vi "Torque Page.vi"(8 "error in (no error)":errorcluster, 11 "Node Ptr":T5 format="%.0x") -> (0 "error out":errorcluster)   [LabVIEW 2010, in "PXIe-433x Custom Device.lvlib"]
uses:
  PXIe-433x Custom Device.lvlib
  <vilib>/NI Veristand/Custom Device API/Custom Device Item Ref.ctl
  Generic Bridge Information.ctl
  Torque Scaling Information.ctl
  Max Value.ctl
  Min Value.ctl
  Board Info for checking settings.ctl
  Scale Type.ctl
  Sensor Type.ctl
  Global.vi
  <vilib>/NI VeriStand/Custom Device API/Get Item Property (Variant).vi
  <vilib>/NI VeriStand/Custom Device API/Get Item Property (Double).vi
  <vilib>/NI Veristand/Custom Device API/Set Item Property (Variant).vi
  <vilib>/NI Veristand/Custom Device API/Set Item Property (Double).vi
  <vilib>/NI Veristand/Custom Device API/Custom Device API.lvlib
panel:
  in  "Board Info for checking":T1
  in  "Minimum Value":T2=-0.05 caption="lb-in"
  in  "Maximum Value":T3=0.05 caption="lb-in"
  out "Error Description":string
  out "Tab Control":enum32{"No Error", "No Check", "Error"}(tab)
  out "Valid":bool=TRUE
  in  "No Error Check Details":bool
  out "No Check":bool=TRUE
  in  "Error Details":bool
  in  "stop":bool
  out "Valid Configuration?":bool
  in  "bridge information":T4={"bridge configuration"=10182, "voltage excitation source"=10200, "voltage excitation value"=2.5, "nominal bridge resistance"=350.0} {"voltage excitation source" items=["Internal"=10200, "External"=10167]; "bridge configuration" items=["Full Bridge"=10182, "Half Bridge"=10187, "Quarter Bridge"=10270]}
  in  "scaling information":T6={"first electrical value"=0.0, "second electrical value"=2.0, "electrical units"=15897, "first physical value"=0.0, "second physical value"=100.0, "physical units"=15883} {"physical units" items=["Nm"=15881, "oz-in"=15882, "lb-in"=15883, "lb-ft"=15884]; "electrical units" items=["Volts/Volt"=15896, "mVolts/Volt"=15897]}
  # "No Error"
  # "No Error"
  # "No Error Check"
  # "No Error Check"
  # "Error!"
  # "Error!"
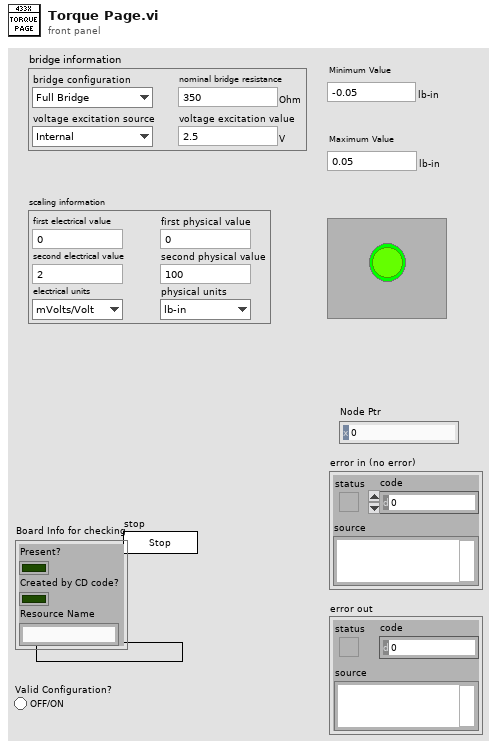
[diagram p1: front panel]
types:
  T1 = typedef "PXIe-433x Custom Device.lvlib/Board Info for checking settings.ctl" = cluster{"Present?":bool, "Created by CD code?":bool, "Resource Name":string}
  T2 = typedef "PXIe-433x Custom Device.lvlib/Min Value.ctl" = dbl
  T3 = typedef "PXIe-433x Custom Device.lvlib/Max Value.ctl" = dbl
  T4 = typedef "PXIe-433x Custom Device.lvlib/Generic Bridge Information.ctl" = cluster{"bridge configuration":i32, "voltage excitation source":i32, "voltage excitation value":dbl, "nominal bridge resistance":dbl}
  T5 = typedef "Custom Device API.lvlib/Custom Device Item Ref.ctl" = u64
  T6 = typedef "PXIe-433x Custom Device.lvlib/Torque Scaling Information.ctl" = cluster{"first electrical value":dbl, "second electrical value":dbl, "electrical units":i32, "first physical value":dbl, "second physical value":dbl, "physical units":i32}
  T7 = typedef "PXIe-433x Custom Device.lvlib/Scale Type.ctl" = enum16{"Linear", "Table", "Polynomial"}
  T8 = typedef "PXIe-433x Custom Device.lvlib/Sensor Type.ctl" = enum16{"Strain", "Force", "Pressure", "Torque"}
  T9 = typedef "Custom Device API.lvlib/Custom Device Commands.ctl" = enum16{"Default", "Item renamed", "Shutdown", "Dynamic button pressed"}
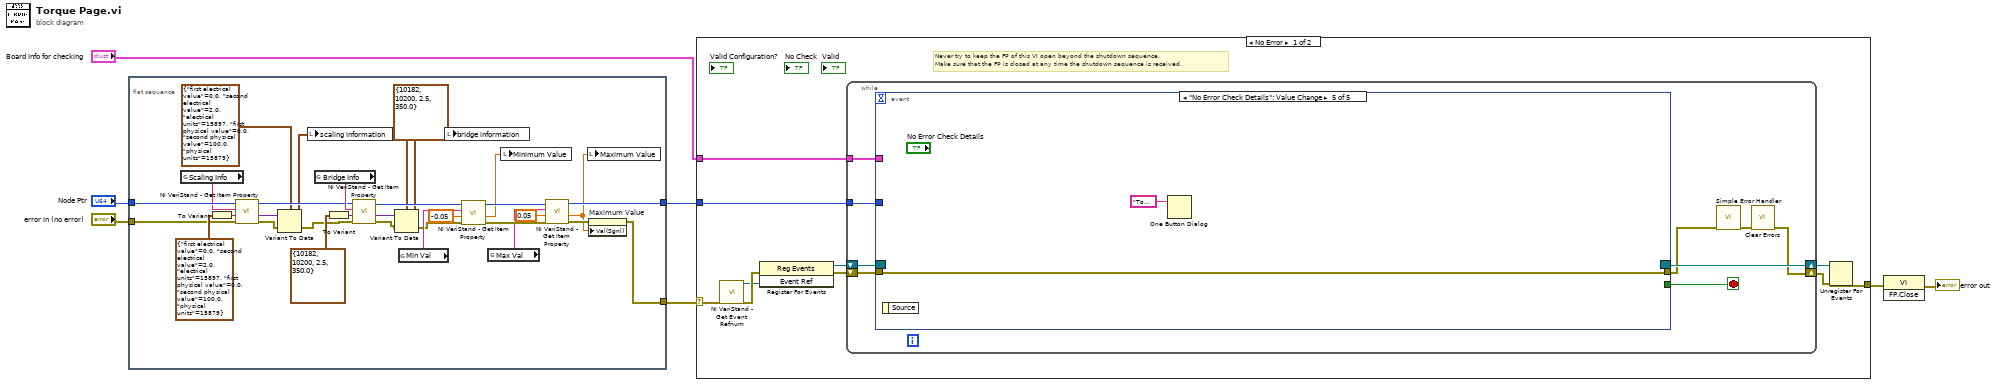
[diagram p0: block diagram]
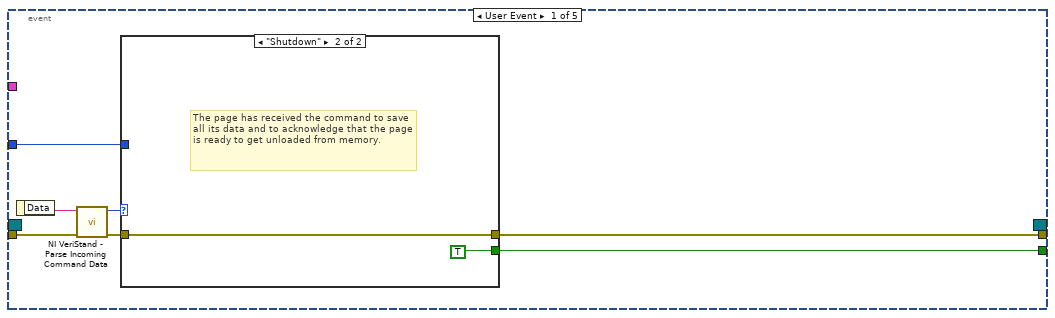
[diagram p2: hidden frame]
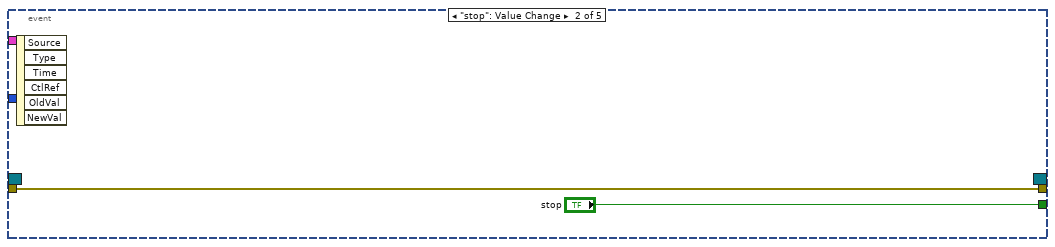
[diagram p4: hidden frame]
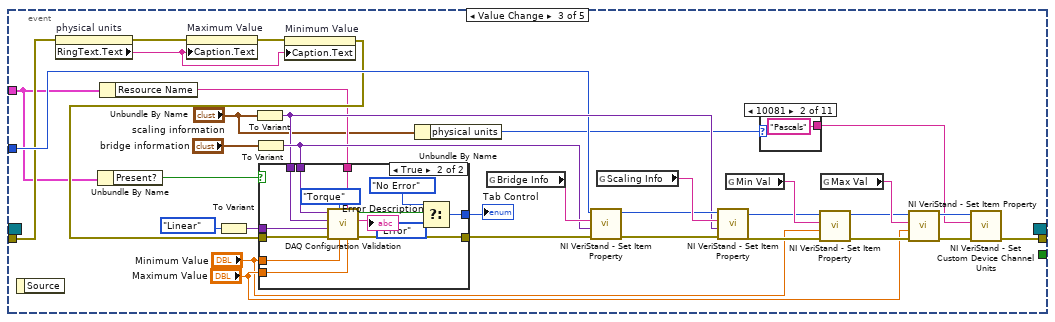
[diagram p5: hidden frame]
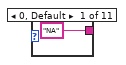
[diagram p6: hidden frame]
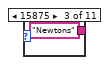
[diagram p7: hidden frame]
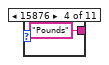
[diagram p8: hidden frame]
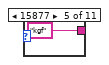
[diagram p9: hidden frame]
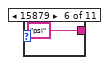
[diagram p10: hidden frame]
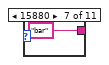
[diagram p11: hidden frame]
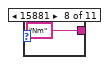
[diagram p12: hidden frame]
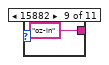
[diagram p13: hidden frame]
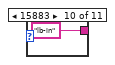
[diagram p14: hidden frame]
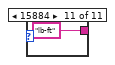
[diagram p15: hidden frame]
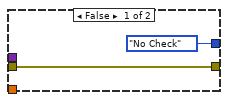
[diagram p16: hidden frame]
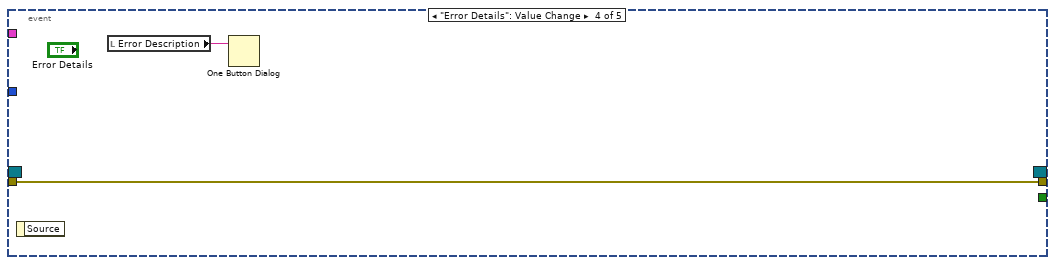
[diagram p17: hidden frame]
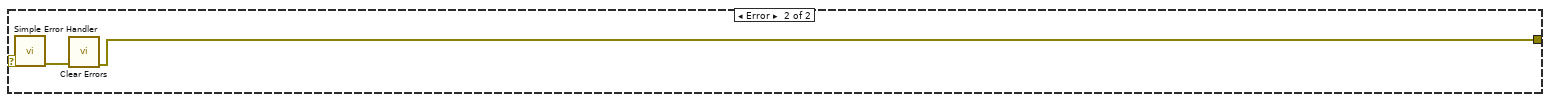
[diagram p18: hidden frame]
diagram:
  n1 = flat-sequence {
    tunnel: [w23] -> w6
    tunnel: "Node Ptr" -> [w38]
    tunnel: [w19] -> w5
    tunnel: "error in (no error)" -> [w8]
    frame #0 {
      n2 = global read "Global.vi" "Scaling Info"() -> (w37:string)
      n3 = To Variant(anything=T6 {"first electrical value"=0.0, "second electrical value"=2.0, "electrical units"=15897, "first physical value"=0.0, "second physical value"=100.0, "physical units"=15879} ("scaling information")) -> (Variant=w36:variant)
      n4 = call-poly <vilib>:"NI VeriStand - Get Item Property.vi"("error in (no error)"=w8, "Default Value"=w36, "Property Name"=w37, "Item Ref in"=w38) -> ("error out"=w16:errorcluster, "Value"=w35:variant, "Item Ref out"=w32:T5)  [unwired: 4 in, 1 out]
      n5 = Variant To Data(error in=w16, Variant=w35, type=T6 {"first electrical value"=0.0, "second electrical value"=2.0, "electrical units"=15897, "first physical value"=0.0, "second physical value"=100.0, "physical units"=15879} ("scaling information")) -> (error out=w15:errorcluster, data=w11:T6)
      n6 = local write "scaling information"(w11) -> ()
      n7 = global read "Global.vi" "Bridge Info"() -> (w34:string)
      n8 = To Variant(anything=T4 {"bridge configuration"=10182, "voltage excitation source"=10200, "voltage excitation value"=2.5, "nominal bridge resistance"=350.0} ("bridge information")) -> (Variant=w30:variant)
      n9 = call-poly <vilib>:"NI VeriStand - Get Item Property.vi"("error in (no error)"=w15, "Default Value"=w30, "Property Name"=w34, "Item Ref in"=w32) -> ("error out"=w14:errorcluster, "Value"=w33:variant, "Item Ref out"=w24:T5)  [unwired: 4 in, 1 out]
      n10 = Variant To Data(error in=w14, Variant=w33, type=T4 {"bridge configuration"=10182, "voltage excitation source"=10200, "voltage excitation value"=2.5, "nominal bridge resistance"=350.0} ("bridge information")) -> (error out=w13:errorcluster, data=w10:T4)
      n11 = global read "Global.vi" "Min Val"() -> (w25:string)
      n12 = local write "bridge information"(w10) -> ()
      n13 = call-poly <vilib>:"NI VeriStand - Get Item Property.vi"("error in (no error)"=w13, "Default Value"=-0.05, "Property Name"=w25, "Item Ref in"=w24) -> ("error out"=w28:errorcluster, "Value"=w27:dbl, "Item Ref out"=w29:T5)  [unwired: 4 in, 1 out]
      n14 = global read "Global.vi" "Max Val"() -> (w26:string)
      n15 = local write "Minimum Value"(w27) -> ()
      n16 = call-poly <vilib>:"NI VeriStand - Get Item Property.vi"("error in (no error)"=w28, "Default Value"=0.05, "Property Name"=w26, "Item Ref in"=w29) -> ("error out"=w20:errorcluster, "Value"=w18:dbl, "Item Ref out"=w23:T5)  [unwired: 4 in, 1 out]
      n17 = local write "Maximum Value"(w18) -> ()
      n18 = property on="Maximum Value" class="DigNum (strict)"(error in=w20, "Val(Sgnl)"=w18) -> (error out=w19:errorcluster)  [unwired: 1 in, 1 out]
    }
  }
  n19 = case shown="No Error" w5 {
    selector: w5 -> [w40 w137]
    tunnel: [w45 w135] -> w7
    tunnel: w6 -> [w41 _]
    tunnel: "Board Info for checking" -> [w39 _]
    frame No Error {
      # "Never try to keep the FP of this VI open beyond the shutdown sequence.\nMake sure that the FP is closed at any time the shutdown sequence is received."
      n20 = call <vilib>:"NI VeriStand - Get Event Refnum.vi"("error in (no error)"=w40) -> ("error out"=w48:errorcluster, "Event Ref"=w44:refnum<user-event>)  [unwired: 9 out]
      n21 = register-events(error in=w48, w44) -> (reference out=w42:refnum<event-registration>, error out=w43:errorcluster)  [unwired: 1 in]
      n22 = while {
        tunnel: w41 -> [w54]
        shift-right: [w51] -> w46
        shift-left: w43 -> [w56]
        shift-right: [w57] -> w47
        shift-left: w42 -> [w55]
        tunnel: w39 -> [w49]
        stop <- w50 stop-if-true
        n23 = event shown="[4] \"No Error Check Details\": Value Change" {
          selector: w55 -> [_ _ _ _ _]
          dyn-events: [_ _ _ _ _] -> w57
          timeout: _ -> [_ _ _ _ _]
          tunnel: w56 -> [w64 w68 w81 w131 w134]
          tunnel: [w60 "stop" _ _ _] -> w50
          tunnel: [w59 w68 w72 w131 w134] -> w53
          tunnel: w54 -> [w58 _ w86 _ _]
          tunnel: w49 -> [_ _ w77 _ _]
          event User Event {
            n24 = event-data() -> ("Data"=w63:string)  [unwired: 1 out]
            n25 = call <vilib>:"NI VeriStand - Parse Incoming Command Data.vi"("error in (no error)"=w64, "Data"=w63) -> ("error out"=w62:errorcluster, "Action"=w61:T9)  [unwired: 8 out]
            n26 = case shown="\"Shutdown\"" w61 {
              tunnel: w62 -> [w65 w66]
              tunnel: [_ TRUE] -> w60
              tunnel: [w65 w66] -> w59
              tunnel: w58 -> [_ _]
              frame "Default", Default {
              }
              frame "Shutdown" {
                # "The page has received the command to save all its data and to acknowledge that the page is ready to get unloaded from memory."
              }
            }
          }
          event "stop": Value Change {
            n27 = event-data() -> ()  [unwired: 7 out]
          }
          event Value Change {
            n28 = event-data() -> ()  [unwired: 2 out]
            n29 = property on="physical units" class="Ring (strict)"(error in=w81) -> (error out=w80:errorcluster, "RingText.Text"=w79:string)  [unwired: 1 in, 1 out]
            n30 = Unbundle By Name(w77) -> ("Present?"=w102:bool)
            n31 = Unbundle By Name(w77) -> ("Resource Name"=w76:string)
            n32 = property on="Maximum Value" class="DigNum (strict)"(error in=w80, "Caption.Text"=w79) -> (error out=w85:errorcluster)  [unwired: 1 in, 1 out]
            n33 = To Variant(anything=Scale_Type."Linear" ("Scale Type")) -> (Variant=w82:variant)
            n34 = To Variant(anything="scaling information") -> (Variant=w95:variant)
            n35 = To Variant(anything="bridge information") -> (Variant=w99:variant)
            n36 = property on="Minimum Value" class="DigNum (strict)"(error in=w85, "Caption.Text"=w79) -> (error out=w84:errorcluster)  [unwired: 1 in, 1 out]
            n37 = case shown="True" w102 {
              tunnel: w84 -> [w116 w130]
              tunnel: [w116 w123] -> w100
              tunnel: "Minimum Value" -> [_ w128]
              tunnel: "Maximum Value" -> [_ w127]
              tunnel: w95 -> [_ w125]
              tunnel: w99 -> [_ w126]
              tunnel: [enum32{"No Error", "No Check", "Error"}."No Check" ("Tab Control") w121] -> w103
              tunnel: w82 -> [_ w118]
              tunnel: w76 -> [_ w117]
              frame False {
              }
              frame True {
                n38 = call "DAQ Configuration Validation.vi"("Maximum Value"=w127, "DAQ Resource Name"=w117, "Minimum Value"=w128, "Sensor Type"=Sensor_Type."Torque", "error in"=w130, "scale type"=w118, "scaling info"=w125, "bridge info"=w126) -> ("error IO"=w123:errorcluster, "Error Source"=→"Error Description":string, "Valid configuration?"=w119:bool)  [unwired: 1 in]
                n39 = Select(t=enum32{"No Error", "No Check", "Error"}."No Error" ("Tab Control"), s=w119, f=enum32{"No Error", "No Check", "Error"}."Error" ("Tab Control")) -> (s? t:f=w121:enum32{"No Error", "No Check", "Error"})
              }
            }
            "Tab Control" <- w103
            n40 = Unbundle By Name("scaling information") -> ("physical units"=w74:i32)
            n41 = global read "Global.vi" "Bridge Info"() -> (w101:string)
            n42 = call-poly <vilib>:"NI VeriStand - Set Item Property.vi"("error in (no error)"=w100, "Value"=w99, "Property Name"=w101, "Item Ref in"=w86) -> ("error out"=w96:errorcluster, "Item Ref out"=w97:T5)  [unwired: 5 in, 1 out]
            n43 = global read "Global.vi" "Scaling Info"() -> (w98:string)
            n44 = call-poly <vilib>:"NI VeriStand - Set Item Property.vi"("error in (no error)"=w96, "Value"=w95, "Property Name"=w98, "Item Ref in"=w97) -> ("error out"=w93:errorcluster, "Item Ref out"=w92:T5)  [unwired: 5 in, 1 out]
            n45 = global read "Global.vi" "Min Val"() -> (w94:string)
            n46 = case shown="10081" w74 {
              tunnel: ["NA" "Pascals" "Newtons" "Pounds" "kgf" "psi" "bar" "Nm" "oz-in" "lb-in" "lb-ft"] -> w70
              frame 0, Default {
              }
              frame 10081 {
              }
              frame 15875 {
              }
              frame 15876 {
              }
              frame 15877 {
              }
              frame 15879 {
              }
              frame 15880 {
              }
              frame 15881 {
              }
              frame 15882 {
              }
              frame 15883 {
              }
              frame 15884 {
              }
            }
            n47 = call-poly <vilib>:"NI VeriStand - Set Item Property.vi"("error in (no error)"=w93, "Value"="Minimum Value", "Property Name"=w94, "Item Ref in"=w92) -> ("error out"=w90:errorcluster, "Item Ref out"=w89:T5)  [unwired: 5 in, 1 out]
            n48 = global read "Global.vi" "Max Val"() -> (w91:string)
            n49 = call-poly <vilib>:"NI VeriStand - Set Item Property.vi"("error in (no error)"=w90, "Value"="Maximum Value", "Property Name"=w91, "Item Ref in"=w89) -> ("error out"=w73:errorcluster, "Item Ref out"=w71:T5)  [unwired: 5 in, 1 out]
            n50 = call <vilib>:"NI VeriStand - Set Custom Device Channel Units.vi"("error in (no error)"=w73, "Units"=w70, "Channel Ref in"=w71) -> ("error out"=w72:errorcluster)  [unwired: 7 in, 1 out]
          }
          event "Error Details": Value Change {
            n51 = event-data() -> ()  [unwired: 2 out]
            n52 = local read "Error Description"() -> (w132:string)
            n53 = One Button Dialog(message=w132) -> ()  [unwired: 1 in, 1 out]
          }
          event "No Error Check Details": Value Change {
            n54 = event-data() -> ()  [unwired: 2 out]
            n55 = One Button Dialog(message="To perform error checking during Edition time, code needs either a physical local PXIe-433x or simulated one. One simulated couldn't be created, no error checking will be performed while editing settings. Error checking will still be performed while deploying Custom-Device.") -> ()  [unwired: 1 in, 1 out]
          }
        }
        n56 = call <vilib>:"Simple Error Handler.vi"("error in (no error)"=w53) -> ("error out"=w52:errorcluster)  [unwired: 1 in, 7 out]
        n57 = call <vilib>:"Clear Errors.vi"("error in (no error)"=w52) -> ("error out"=w51:errorcluster)  [unwired: 6 out]
      }
      n58 = Unregister For Events(event registration refnum=w47, error in=w46) -> (error out=w45:errorcluster)
    }
    frame Error {
      n59 = call <vilib>:"Simple Error Handler.vi"("error in (no error)"=w137) -> ("error out"=w136:errorcluster)  [unwired: 1 in, 7 out]
      n60 = call <vilib>:"Clear Errors.vi"("error in (no error)"=w136) -> ("error out"=w135:errorcluster)  [unwired: 6 out]
    }
  }
  n61 = invoke class="VI" method="FP.Close"(error in=w7) -> (error out=→"error out":errorcluster)  [unwired: 2 in, 2 out]
